vi "Recognize Text.vi"   [LabVIEW 2020, in "feature_detection.lvlib" / "Text Recognizer.lvclass"]
uses:
  Text Recognizer.lvclass
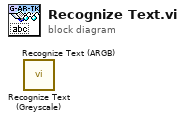
[diagram p0: block diagram]
diagram:
  n1 = call "Recognize Text (Greyscale).vi"() -> ()  [unwired: 9 in, 3 out]
  n2 = call "Recognize Text (ARGB).vi"() -> ()  [unwired: 9 in, 3 out]
